vi "get_rpm_WinAvg.vi"(2 "error in (no error)":errorcluster) -> (0 "RPM":dbl, 1 "error out":errorcluster)   [LabVIEW 2019]
uses:
  rpm.vi
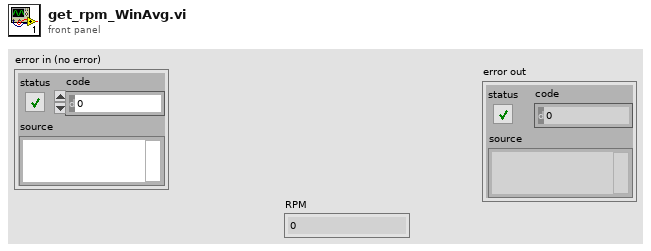
[diagram p1: front panel]
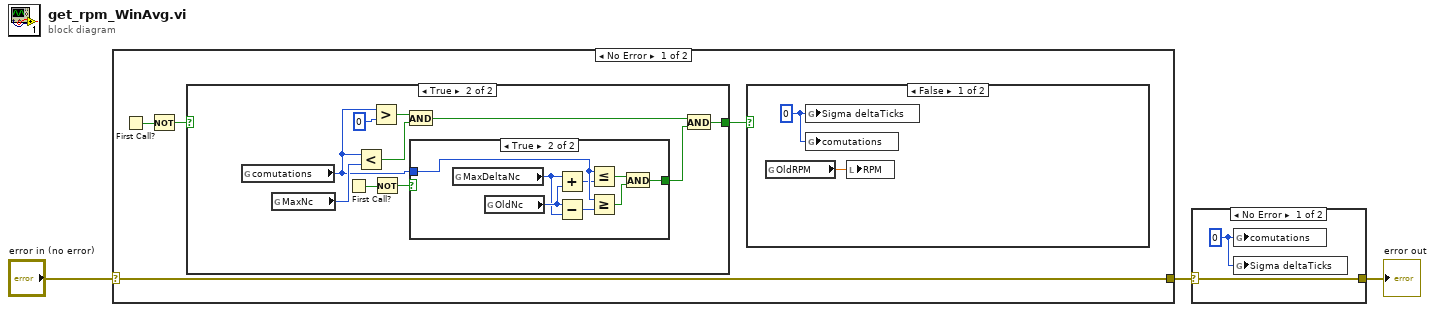
[diagram p0: block diagram]
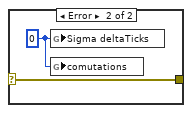
[diagram p2: hidden frame]
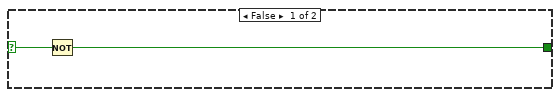
[diagram p3: hidden frame]
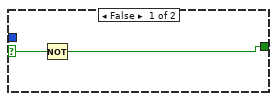
[diagram p4: hidden frame]
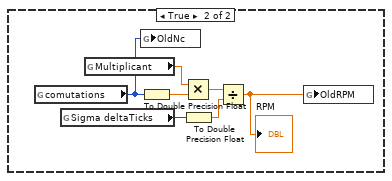
[diagram p5: hidden frame]
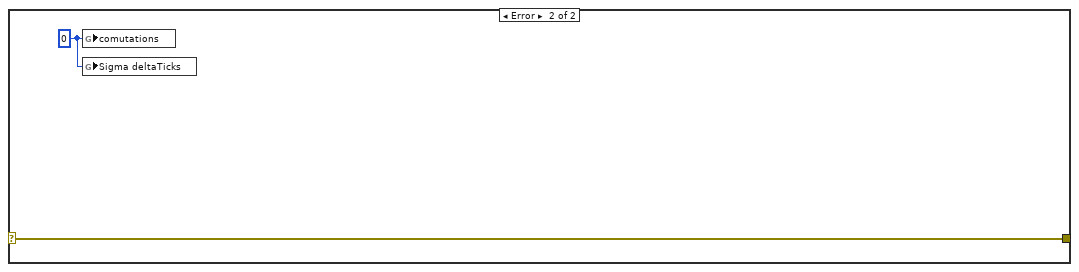
[diagram p6: hidden frame]
diagram:
  n1 = case shown="No Error" "error in (no error)" {
    selector: "error in (no error)" -> [w7 w40]
    tunnel: [w7 w40] -> w3
    frame No Error {
      n2 = First Call?() -> (First Call?: T/F=w5:bool)
      n3 = Not(x=w5) -> (.not. x?=w4:bool)
      n4 = case shown="True" w4 {
        selector: w4 -> [w9 _]
        tunnel: [w8 w15] -> w6
        frame False {
          n5 = Not(x=w9) -> (.not. x?=w8:bool)
        }
        frame True {
          n6 = global read "rpm.vi" "comutations"() -> (w13:i64)
          n7 = global read "rpm.vi" "MaxNc"() -> (w16:i64)
          n8 = First Call?() -> (First Call?: T/F=w11:bool)
          n9 = Less?(x=w13, y=w16) -> (x < y?=w17:bool)
          n10 = Greater?(x=w13, y=i64 0) -> (0:w18:bool)
          n11 = Not(x=w11) -> (.not. x?=w10:bool)
          n12 = And(x=w18, y=w17) -> (x .and. y?=w14:bool)
          n13 = case shown="True" w10 {
            selector: w10 -> [w21 _]
            tunnel: w13 -> [_ w29]
            tunnel: [w20 w28] -> w12
            frame False {
              n14 = Not(x=w21) -> (.not. x?=w20:bool)
            }
            frame True {
              n15 = global read "rpm.vi" "MaxDeltaNc"() -> (w22:i64)
              n16 = global read "rpm.vi" "OldNc"() -> (w23:i64)
              n17 = Add(x=w22, y=w23) -> (x+y=w25:i64)
              n18 = Subtract(x=w23, y=w22) -> (x-y=w24:i64)
              n19 = Less Or Equal?(x=w29, y=w25) -> (x <= y?=w26:bool)
              n20 = Greater Or Equal?(x=w29, y=w24) -> (x >= y?=w27:bool)
              n21 = And(x=w26, y=w27) -> (x .and. y?=w28:bool)
            }
          }
          n22 = And(x=w14, y=w12) -> (x .and. y?=w15:bool)
        }
      }
      n23 = case shown="False" w6 {
        frame False {
          w30 = i64 0 ("comutations")
          n24 = global read "rpm.vi" "OldRPM"() -> (w31:dbl)
          n25 = global write "rpm.vi" "Sigma deltaTicks"(w30) -> ()
          n26 = global write "rpm.vi" "comutations"(w30) -> ()
          n27 = local write "RPM"(w31) -> ()
        }
        frame True {
          n28 = global read "rpm.vi" "comutations"() -> (w32:i64)
          n29 = global read "rpm.vi" "Sigma deltaTicks"() -> (w38:i64)
          n30 = global read "rpm.vi" "Multiplicant"() -> (w36:dbl)
          n31 = global write "rpm.vi" "OldNc"(w32) -> ()
          n32 = To Double Precision Float(number=w32) -> (double precision float=w37:dbl)
          n33 = Multiply(x=w36, y=w37) -> (x*y=w35:dbl)
          n34 = To Double Precision Float(number=w38) -> (double precision float=w34:dbl)
          n35 = Divide(x=w35, y=w34) -> (x/y=w33:dbl)
          "RPM" <- w33
          n36 = global write "rpm.vi" "OldRPM"(w33) -> ()
        }
      }
    }
    frame Error {
      w39 = i64 0 ("comutations")
      n37 = global write "rpm.vi" "comutations"(w39) -> ()
      n38 = global write "rpm.vi" "Sigma deltaTicks"(w39) -> ()
    }
  }
  n39 = case shown="No Error" w3 {
    selector: w3 -> [w42 w44]
    tunnel: [w42 w44] -> w1
    frame No Error {
      w41 = i64 0 ("comutations")
      n40 = global write "rpm.vi" "comutations"(w41) -> ()
      n41 = global write "rpm.vi" "Sigma deltaTicks"(w41) -> ()
    }
    frame Error {
      w43 = i64 0 ("comutations")
      n42 = global write "rpm.vi" "Sigma deltaTicks"(w43) -> ()
      n43 = global write "rpm.vi" "comutations"(w43) -> ()
    }
  }
  "error out" <- w1
